vi "Read All Memory Values.vi"(8 "error in (no error)":errorcluster, 11 "VISA resource name":refnum<visa-resource-name>) -> (0 "error out":errorcluster, 3 "VISA resource name out":refnum<visa-resource-name>)   [LabVIEW 2021, in "BK Precision 169XB.lvlib"]
doc: "Returns the actual voltage level and actual current level for a desired channel."
uses:
  BK Precision 169XB.lvlib
panel:
  out "Current":dbl[](array[numeric]) format="%.2g"
  out "Voltage":dbl[](array[numeric]) format="%.1g"
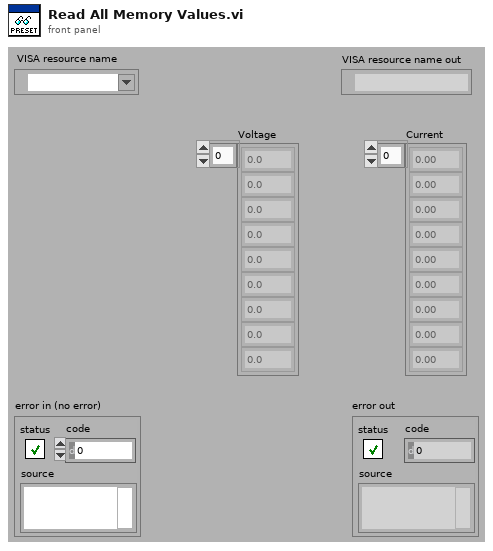
[diagram p1: front panel]
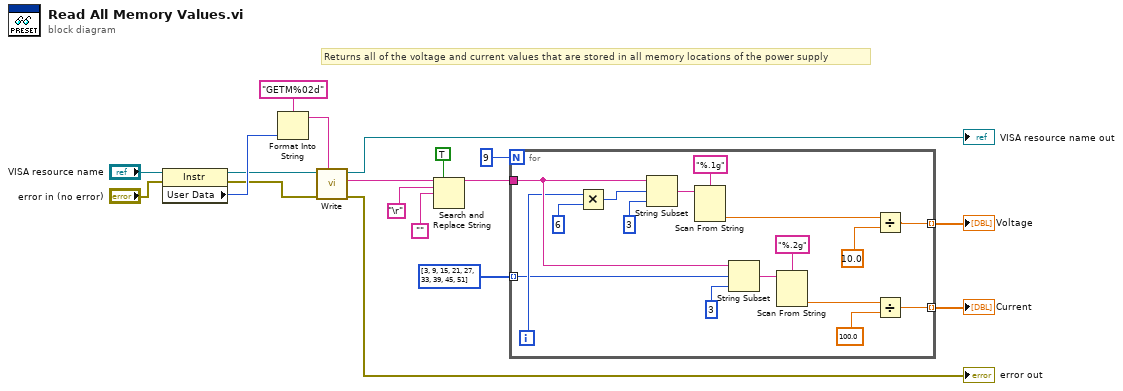
[diagram p0: block diagram]
diagram:
  # "Returns all of the voltage and current values that are stored in all memory locations of the power supply"
  n1 = property class="Instr"(reference="VISA resource name", error in="error in (no error)") -> (reference out=w10:refnum<visa-resource-name>, error out=w7:errorcluster, "User Data"=w12:u32)
  n2 = Format Into String(format string="GETM%02d", w12) -> (resulting string=w9:string)  [unwired: 2 in, 1 out]
  n3 = call "Write.vi"("Input String"=w9, "error in (no error)"=w7, "VISA resource name"=w10) -> ("error out"=→"error out":errorcluster, "String"=w6:string, "VISA resource name out"=→"VISA resource name out":refnum<visa-resource-name>)  [unwired: 6 in]
  n4 = Search and Replace String(replace all?=TRUE ("replace all? (F)"), input string=w6, search string="\r", replace string="") -> (result string=w5:string)  [unwired: 4 in, 3 out]
  n5 = for {
    N: 9 -> [_]
    tunnel: w5 -> [w29]
    tunnel: [w26] -> w15 mode=indexing
    tunnel: [w24] -> w14 mode=indexing
    tunnel: i32[] [3, 9, 15, 21, 27, 33, 39, 45, 51] -> [w19] mode=indexing
    i -> [w28]
    n6 = Multiply(x=w28, y=6) -> (x*y=w33:i32)
    n7 = String Subset(string=w29, offset (0)=w33, length (rest)=3 ("length (rest)")) -> (substring=w32:string)
    n8 = Scan From String(format string="%.1g", input string=w32) -> (output 1=w27:dbl)  [unwired: 3 in, 3 out]
    n9 = String Subset(string=w29, offset (0)=w19, length (rest)=3 ("length (rest)")) -> (substring=w31:string)
    n10 = Scan From String(format string="%.2g", input string=w31) -> (output 1=w25:dbl)  [unwired: 3 in, 3 out]
    n11 = Divide(x=w27, y=10.0) -> (x/y=w26:dbl)
    n12 = Divide(x=w25, y=100.0) -> (x/y=w24:dbl)
  }
  "Voltage" <- w15
  "Current" <- w14
